vi "NIRepToRGB.vi"(0 "color":u32(colorbox)) -> (1 "red":u8, 2 "green":u8, 3 "blue":u8, 4 "transparent?":bool)   [LabVIEW 2015, in "NI_ReportGenerationCore.lvlib"]
doc: "Non-API VI."
uses:
  <vilib>/Utility/NIReport.llb/NI_ReportGenerationCore.lvlib
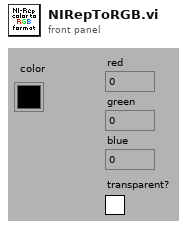
[diagram p1: front panel]
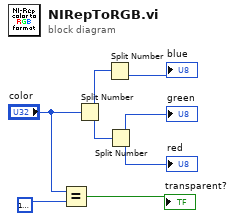
[diagram p0: block diagram]
diagram:
  n1 = Equal?(x="color", y=u32 16777216 ("color")) -> (x = y?=→"transparent?":bool)
  n2 = Split Number(x="color") -> (hi(x)=w4:u16, lo(x)=w3:u16)
  n3 = Split Number(x=w4) -> (lo(x)=→"blue":u8)  [unwired: 1 out]
  n4 = Split Number(x=w3) -> (hi(x)=→"green":u8, lo(x)=→"red":u8)
